vi "IMAQ FPGA Camera Link Data to Pixels 2 Tap 10-Bit.vi"(1 "Camera Link Data":cluster{"Port A":u8, "Port B":u8, "Port C":u8}) -> (0 "Pixels":u16[](array[numeric]))   [LabVIEW 2020]
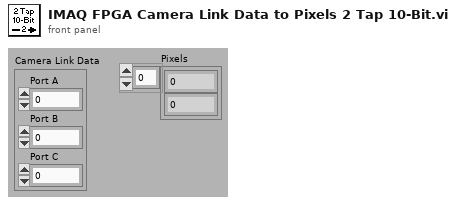
[diagram p1: front panel]
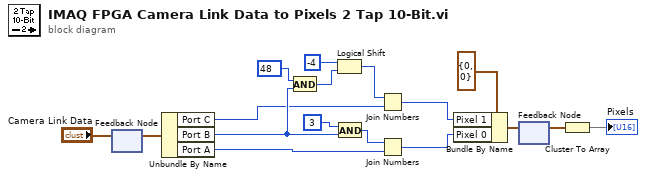
[diagram p0: block diagram]
diagram:
  n1 = feedback-in #1("Camera Link Data") -> ()
  n2 = feedback #1() -> (w3:cluster{"Port A":u8, "Port B":u8, "Port C":u8})  [unwired: 1 in]
  n3 = Unbundle By Name(w3) -> ("Port C"=w5:u8, "Port B"=w6:u8, "Port A"=w7:u8)
  n4 = And(x=u8 48 ("hi"), y=w6) -> (x .and. y?=w13:u8)
  n5 = Logical Shift(y=i8 -4, x=w13) -> (x << y=w11:u8)
  n6 = And(x=u8 3 ("hi"), y=w6) -> (x .and. y?=w15:u8)
  n7 = Join Numbers(hi=w11, lo=w5) -> ((hi.lo)=w9:u16)
  n8 = Join Numbers(hi=w15, lo=w7) -> ((hi.lo)=w10:u16)
  n9 = Bundle By Name(cluster=cluster{"Pixel 0":u16, "Pixel 1":u16} {"Pixel 0"=0, "Pixel 1"=0} ("PixelData"), "Pixel 1"=w9, "Pixel 0"=w10) -> (w2:cluster{"Pixel 0":u16, "Pixel 1":u16})
  n10 = feedback #2() -> (w1:cluster{"Pixel 0":u16, "Pixel 1":u16})  [unwired: 1 in]
  n11 = feedback-in #2(w2) -> ()
  n12 = Cluster To Array(cluster=w1) -> (array=→"Pixels":u16[])
